vi "add server.vi"() -> (0 "Server Array":string[](array[string]), 1 "Server list":string)   [LabVIEW 2012]
uses:
  Process Controller 3.0/read-write.ctl
  Process Controller 3.0/ini interface.ctl
panel:
  in  "Cancel Button":bool
  in  "OK Button":bool
  in  "Server address":string
  # "Edit the computer addresses"
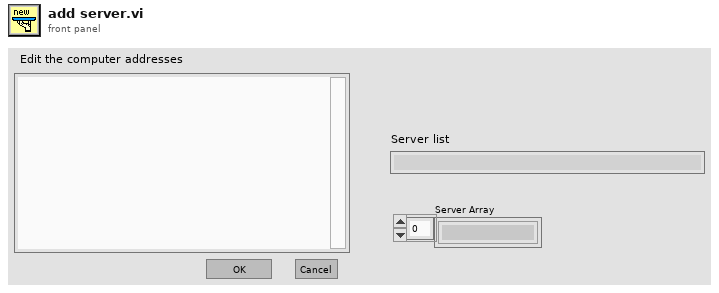
[diagram p1: front panel]
types:
  T1 = typedef "ini interface.ctl" = enum16{"dataserver list", "dataserver", "com port", "stamp model", "Local Daq"}
  T2 = typedef "read-write.ctl" = enum16{"read", "write"}
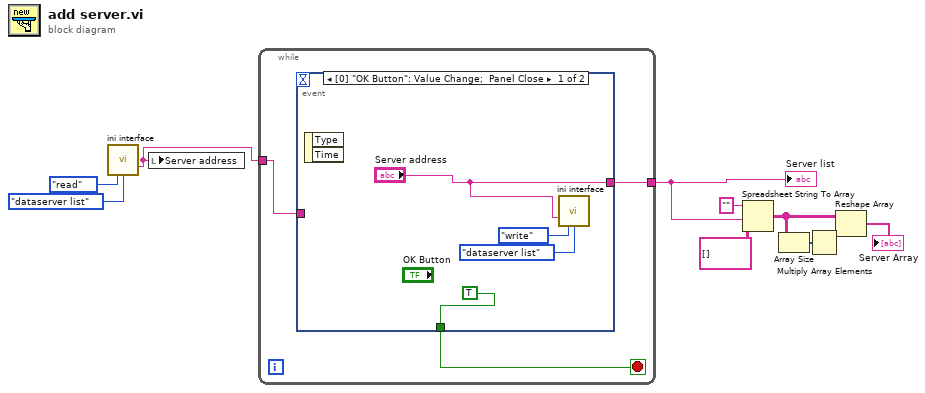
[diagram p0: block diagram]
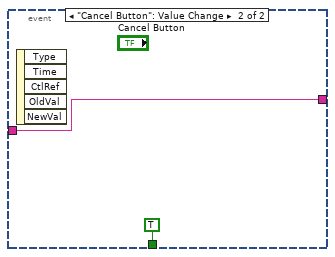
[diagram p2: hidden frame]
diagram:
  n1 = call "ini interface.vi"("direction"=read-write."read", "ini interface"=ini_interface."dataserver list") -> ("dataserver list out"=w8:string)  [unwired: 9 in, 4 out]
  n2 = local write "Server address"(w8) -> ()
  n3 = while {
    tunnel: [w12] -> w2
    tunnel: w8 -> [w11]
    stop <- w13 stop-if-true
    n4 = event shown="[0] \"OK Button\": Value Change;  Panel Close" {
      selector: _ -> [_ _]
      dyn-events: _ -> [_ _]
      timeout: _ -> [_ _]
      tunnel: [TRUE ("OK Button") TRUE ("OK Button")] -> w13
      tunnel: ["Server address" w19] -> w12
      tunnel: w11 -> [_ w19]
      event "OK Button": Value Change; Panel Close {
        n5 = event-data() -> ()  [unwired: 1 in, 2 out]
        n6 = call "ini interface.vi"("dataserver list"="Server address", "direction"=read-write."write", "ini interface"=ini_interface."dataserver list") -> ()  [unwired: 8 in, 5 out]
      }
      event "Cancel Button": Value Change {
        n7 = event-data() -> ()  [unwired: 1 in, 5 out]
      }
    }
  }
  "Server list" <- w2
  n8 = Spreadsheet String To Array(format string="", spreadsheet string=w2, array type (2D Dbl)=string[][] []) -> (array=w4:string[][])  [unwired: 1 in]
  n9 = Array Size(array=w4) -> (size(s)=w3:i32[])
  n10 = Multiply Array Elements(1:w3) -> (0:w7:i32)
  n11 = Reshape Array(w4, w7) -> (→"Server Array":string[])
